vi "Animation State.vi"(10 "Running?":bool, 11 "Function":T1) -> (2 "Running?":bool)   [LabVIEW 2020, in "LMH-Toolbox.lvlib" / "LMH GUI Tools.lvlib"]
uses:
  LMH GUI Tools.lvlib
  Type Defs/Animation FGV State.ctl
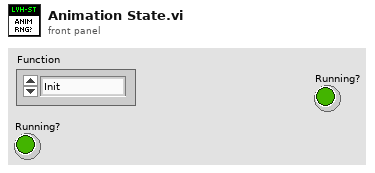
[diagram p1: front panel]
types:
  T1 = typedef "LMH-Toolbox.lvlib/LMH GUI Tools.lvlib/Animation FGV State.ctl" = enum16{"Init", "Set", "Get"}
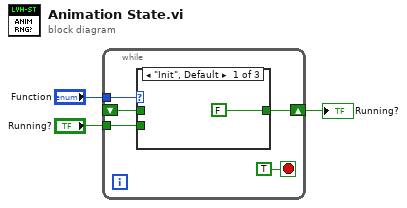
[diagram p0: block diagram]
diagram:
  n1 = while {
    tunnel: "Function" -> [w8]
    shift-right: [w6] -> w2
    shift-left: _ -> [w7]
    tunnel: "Running?" -> [w5]
    stop <- TRUE stop-if-true
    n2 = case shown="\"Init\", Default" w8 {
      tunnel: [FALSE w10 w11] -> w6
      tunnel: w7 -> [_ _ w11]
      tunnel: w5 -> [_ w10 _]
      frame "Init", Default {
      }
      frame "Set" {
      }
      frame "Get" {
      }
    }
  }
  "Running?" <- w2
